vi "background worker.vi"(11 "starburst in":refnum<class "publisher.lvclass">) -> ()   [LabVIEW 2015, in "publisher.lvclass"]
uses:
  publisher.lvclass
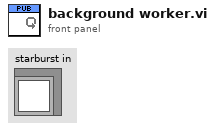
[diagram p1: front panel]
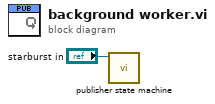
[diagram p0: block diagram]
diagram:
  n1 = call "publisher state machine.vi"("starburst in"="starburst in") -> ()  [unwired: 11 in]
